vi "MakePath.vi"(0 "Numeric":i32, 1 "Path":path) -> (2 "TDMS":path, 3 "BIN":path, 4 "AVI":path)   [LabVIEW 2018]
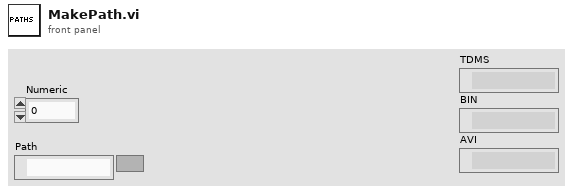
[diagram p1: front panel]
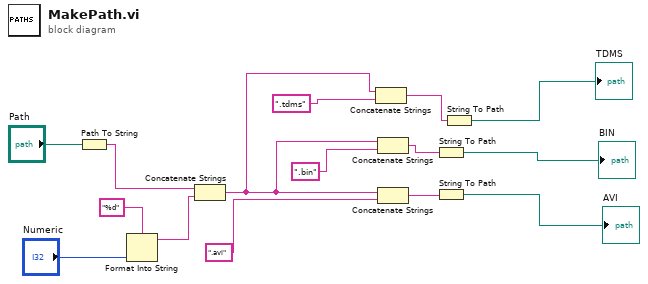
[diagram p0: block diagram]
diagram:
  n1 = Path To String(path="Path") -> (string=w7:string)
  n2 = Format Into String(format string="%d", "Numeric") -> (resulting string=w10:string)  [unwired: 2 in, 1 out]
  n3 = Concatenate Strings(w7, w10) -> (w2:string)
  n4 = Concatenate Strings(w2, ".tdms") -> (w13:string)
  n5 = Concatenate Strings(w2, ".bin") -> (w14:string)
  n6 = Concatenate Strings(w2, ".avi") -> (w15:string)
  n7 = String To Path(string=w14) -> (path=→"BIN":path)
  n8 = String To Path(string=w15) -> (path=→"AVI":path)
  n9 = String To Path(string=w13) -> (path=→"TDMS":path)
